vi "Apply Arc Velocity to Wheels.vi"(5 "wheel indexes":i32[](array[numeric]), 6 "constraint error tolerance (1E-12)":dbl=1e-12, 7 "apply data to motors (F)":bool, 8 "error in (no error)":errorcluster, 10 "arc velocity":T1={"turning radius"=1.0, "tangential velocity"=0.0, "angle from tangent (rad)"=0.0}, 11 "steering frame in":refnum<class "NI_Robotics_Steering Frame.lvclass">) -> (0 "error out":errorcluster, 1 "calculated wheel states":T2[](array[typedef]), 2 "coerced arc velocity":T1={"turning radius"=1.0, "tangential velocity"=0.0, "angle from tangent (rad)"=0.0}, 3 "steering frame out":refnum<class "NI_Robotics_Steering Frame.lvclass">)   [LabVIEW 2017, in "NI_Robotics_Steering Frame.lvclass"]
doc: "Calculates the state of each wheel necessary to satisfy the <B>steering frame velocity</B> or <B>arc velocity</B> at the center of the steering frame. You must manually select the polymorphic instance to use."
uses:
  <vilib>/robotics/Steering/Steering Frame/NI_Robotics_Steering Frame.lvclass
  <vilib>/robotics/Steering/Wheel/Wheel State.ctl
  <vilib>/robotics/Steering/Steering Frame/Arc Velocity.ctl
  <vilib>/robotics/Steering/Wheel/NI_Robotics_Wheel.lvclass
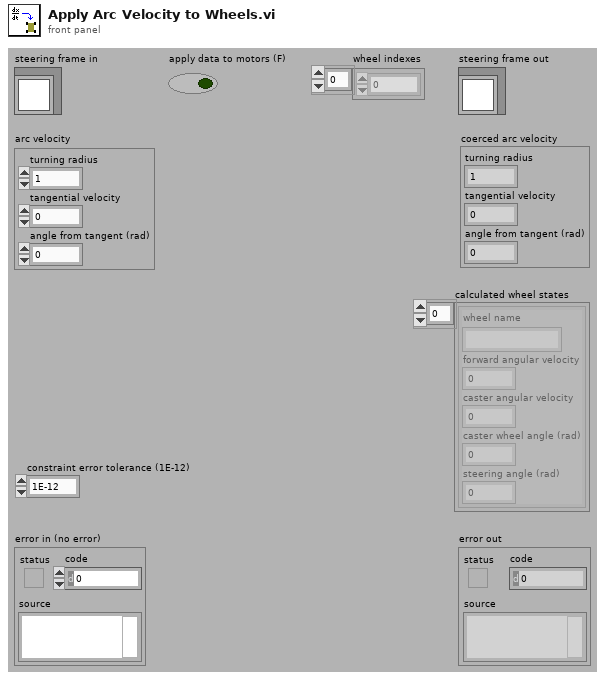
[diagram p1: front panel]
types:
  T1 = typedef "NI_Robotics_Steering Frame.lvclass/Arc Velocity.ctl" = cluster{"turning radius":dbl, "tangential velocity":dbl, "angle from tangent (rad)":dbl}
  T2 = typedef "NI_Robotics_Wheel.lvclass/Wheel State.ctl" = cluster{"wheel name":string, "forward angular velocity":dbl, "caster angular velocity":dbl, "caster wheel angle (rad)":dbl, "steering angle (rad)":dbl}
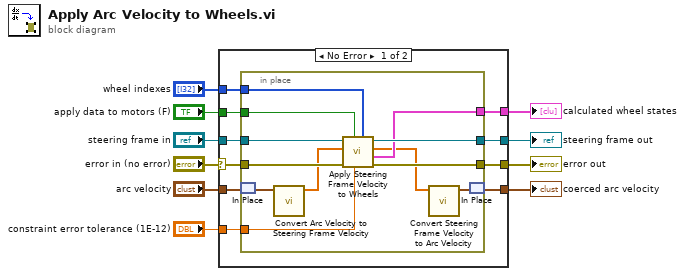
[diagram p0: block diagram]
diagram:
  n1 = case shown="No Error" "error in (no error)" {
    selector: "error in (no error)" -> [w16 w34]
    tunnel: [w15 w34] -> w9
    tunnel: [w19 w33] -> w7
    tunnel: "steering frame in" -> [w20 w33]
    tunnel: "apply data to motors (F)" -> [w18 _]
    tunnel: "constraint error tolerance (1E-12)" -> [w14 _]
    tunnel: [w17 _] -> w4
    tunnel: "arc velocity" -> [w13 _]
    tunnel: [w12 _] -> w2
    tunnel: "wheel indexes" -> [w11 _]
    frame No Error {
      n2 = in-place {
        in-place-border: w20 -> [w32]
        in-place-border: [w31] -> w19
        in-place-border: w18 -> [w30]
        in-place-border: [w29] -> w17
        in-place-border: w16 -> [w28]
        in-place-border: [w27] -> w15
        in-place-border: w14 -> [w24]
        in-place-border: w11 -> [w21]
        n3 = in-place-match #1(w13) -> (w23:T1)
        n4 = call <vilib>:"Convert Arc Velocity to Steering Frame Velocity.vi"("arc velocity"=w23) -> ("steering frame velocity"=w26:dbl[])  [unwired: 10 in]
        n5 = call <vilib>:"Apply Steering Frame Velocity to Wheels.vi"("wheel indexes"=w21, "constraint error tolerance (1E-12)"=w24, "apply data to motors (F)"=w30, "error in (no error)"=w28, "steering frame velocity"=w26, "steering frame in"=w32) -> ("error out"=w27:errorcluster, "calculated wheel states"=w29:T2[], "coerced steering frame velocity"=w25:dbl[], "steering frame out"=w31:refnum<class "NI_Robotics_Steering Frame.lvclass">)  [unwired: 2 in]
        n6 = call <vilib>:"Convert Steering Frame Velocity to Arc Velocity.vi"("steering frame velocity"=w25) -> ("arc velocity"=w22:T1)  [unwired: 10 in]
        n7 = in-place-match #1(w22) -> (w12:T1)
      }
    }
    frame Error {
    }
  }
  "error out" <- w9
  "steering frame out" <- w7
  "calculated wheel states" <- w4
  "coerced arc velocity" <- w2
